vi "recipeScript resizeParamTab.vi"(8 "error in (no error)":errorcluster, 10 "dialogueTopSpl":refnum<vi>, 11 "Parameter Tab":refnum<vi>) -> (0 "error out":errorcluster)   [LabVIEW 2018]
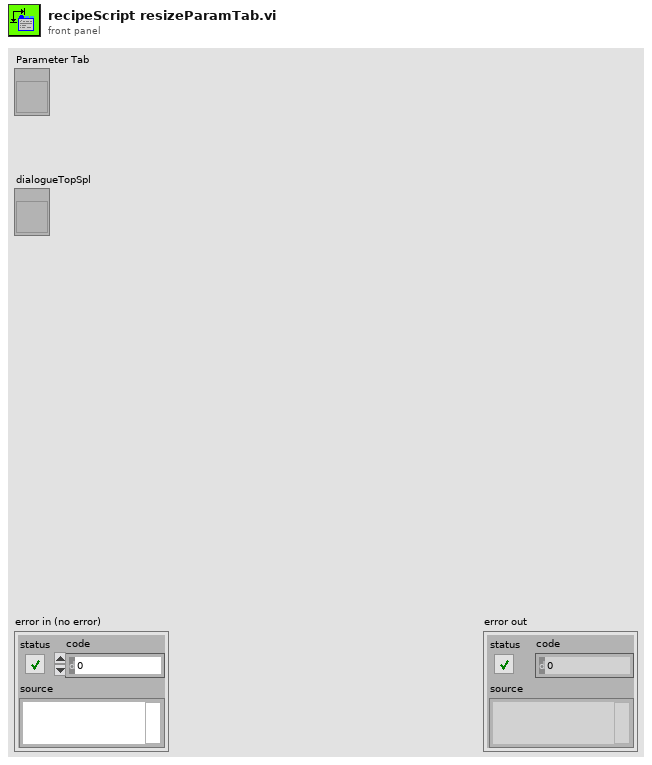
[diagram p1: front panel]
types:
  T1 = enum16{"No Scaling", "Scale All Objects", "Scale Single Object"}
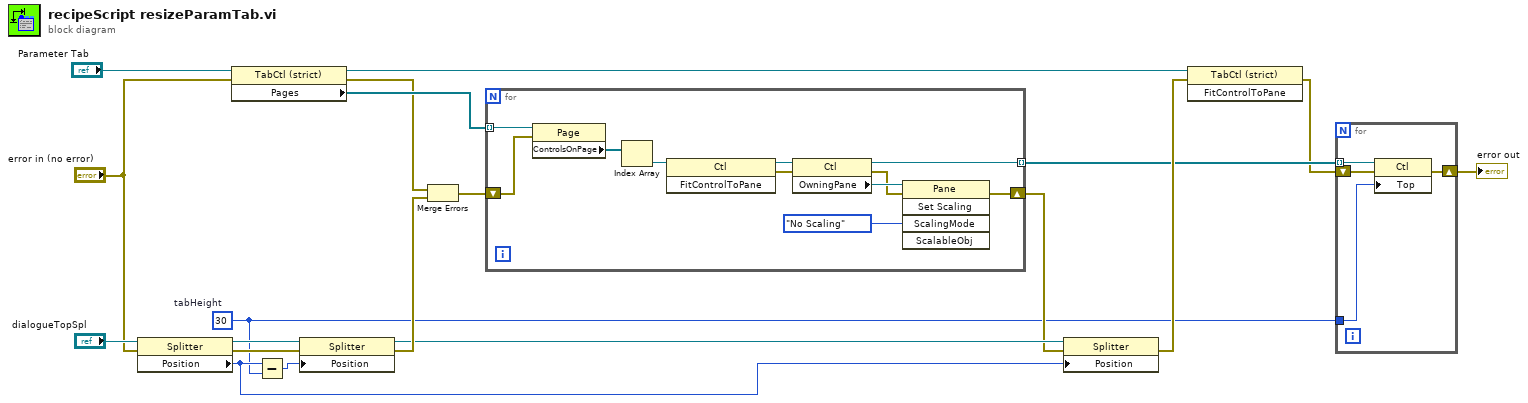
[diagram p0: block diagram]
diagram:
  w3 = 30  # tabHeight
  n1 = property class="Splitter"(reference="dialogueTopSpl", error in="error in (no error)") -> (reference out=w17:refnum<vi>, error out=w16:errorcluster, "Position"=w9:i32)
  n2 = property class="TabCtl (strict)"(reference="Parameter Tab", error in="error in (no error)") -> (reference out=w7:refnum<vi>, error out=w13:errorcluster, "Pages"=w19:refnum<vi>[])
  n3 = Subtract(x=w9, y=w3) -> (x-y=w18:i32)
  n4 = property class="Splitter"(reference=w17, error in=w16, "Position"=w18) -> (reference out=w10:refnum<vi>, error out=w12:errorcluster)
  n5 = Merge Errors(w13, w12) -> (w11:errorcluster)
  n6 = for {
    tunnel: w19 -> [w25] mode=indexing
    tunnel: [w21] -> w5 mode=indexing
    shift-right: [w20] -> w8
    shift-left: w11 -> [w22]
    n7 = property class="Page"(reference=w25, error in=w22) -> ("ControlsOnPage"=w24:refnum<vi>[])  [unwired: 2 out]
    n8 = Index Array(array=w24) -> (element=w23:refnum<vi>)  [unwired: 1 in]
    n9 = invoke class="Ctl" method="FitControlToPane"(reference=w23) -> (reference out=w27:refnum<vi>, error out=w26:errorcluster)  [unwired: 2 in, 1 out]
    n10 = property class="Ctl"(reference=w27, error in=w26) -> (reference out=w21:refnum<vi>, error out=w28:errorcluster, "OwningPane"=w30:refnum<vi>)
    n11 = invoke class="Pane" method="Set Scaling"(reference=w30, error in=w28, "ScalingMode"=T1."No Scaling" ("Scaling Mode")) -> (error out=w20:errorcluster)  [unwired: 2 in, 4 out]
  }
  n12 = property class="Splitter"(reference=w10, error in=w8, "Position"=w9) -> (error out=w6:errorcluster)  [unwired: 1 out]
  n13 = invoke class="TabCtl (strict)" method="FitControlToPane"(reference=w7, error in=w6) -> (error out=w4:errorcluster)  [unwired: 1 in, 2 out]
  n14 = for {
    tunnel: w5 -> [w34] mode=indexing
    tunnel: w3 -> [w32]
    shift-right: [w31] -> w2
    shift-left: w4 -> [w33]
    n15 = property class="Ctl"(reference=w34, error in=w33, "Top"=w32) -> (error out=w31:errorcluster)  [unwired: 1 out]
  }
  "error out" <- w2
